vi "KH7008 Create Command String.vi"(8 "error in (no error)":errorcluster, 11 "Channel Params":T1={"Channel"=enum."Channel 2", "Gain"=enum."10x", "Bandwidth Filter"=enum."ON", "Shunt Resistor"=enum."50 Ohms", "Coupling"=enum."DC", "Input Config"=enum."Differential"}) -> (0 "error out":errorcluster, 3 "Command string":string)   [LabVIEW 2019, in "Inst.Krohn-Hite-7008.lvclass"]
uses:
  Inst.Krohn-Hite-7008.lvclass
  Typedefs/SetAll-Cluster.ctl
  Typedefs/Channel-Enum.ctl
  Typedefs/Gain-Enum.ctl
  Typedefs/Filter-Enum.ctl
  Typedefs/Shunt-Enum.ctl
  Typedefs/Coupling-Enum.ctl
  Typedefs/Input Configuration-Enum.ctl
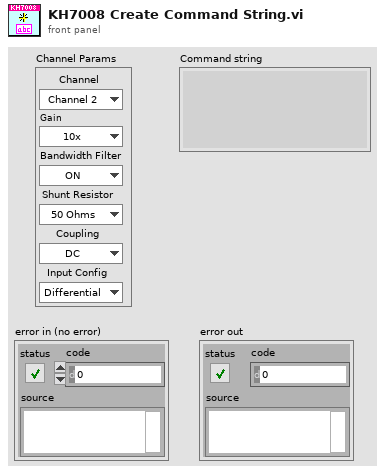
[diagram p1: front panel]
types:
  T1 = typedef "Inst.Krohn-Hite-7008.lvclass/SetAll-Cluster.ctl" = cluster{"Channel":T2, "Gain":T3, "Bandwidth Filter":T4, "Shunt Resistor":T5, "Coupling":T6, "Input Config":T7}
  T2 = typedef "Inst.Krohn-Hite-7008.lvclass/Channel-Enum.ctl" = enum16{"Channel 1", "Channel 2", "Channel 3", "Channel 4", "Channel 5", "Channel 6", "Channel 7", "Channel 8"}
  T3 = typedef "Inst.Krohn-Hite-7008.lvclass/Gain-Enum.ctl" = enum16{"1x", "10x", "100x", "1000x"}
  T4 = typedef "Inst.Krohn-Hite-7008.lvclass/Filter-Enum.ctl" = enum16{"OFF", "ON"}
  T5 = typedef "Inst.Krohn-Hite-7008.lvclass/Shunt-Enum.ctl" = enum16{"Open", "50 Ohms", "500 Ohms", "5k Ohms", "50k Ohms", "10M Ohm"}
  T6 = typedef "Inst.Krohn-Hite-7008.lvclass/Coupling-Enum.ctl" = enum16{"AC", "DC"}
  T7 = typedef "Inst.Krohn-Hite-7008.lvclass/Input Configuration-Enum.ctl" = enum16{"Ground", "SE+ (-gnd)", "SE- (+gnd)", "Differential"}
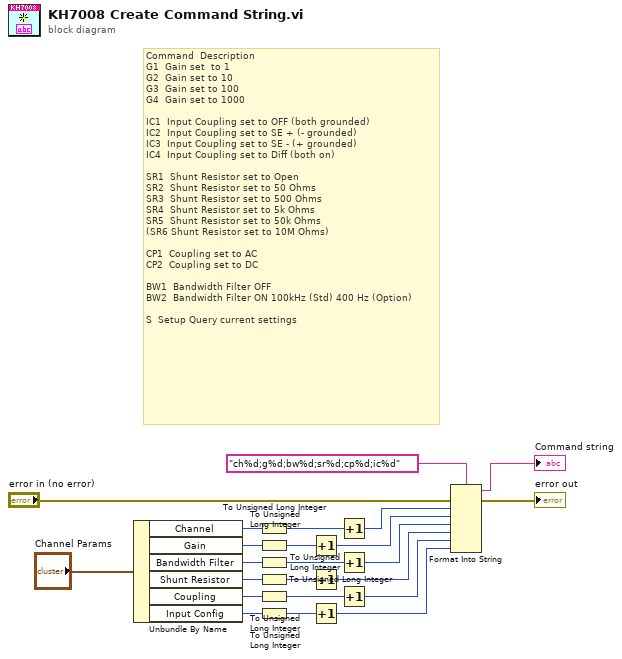
[diagram p0: block diagram]
diagram:
  # "Command  Description \nG1  Gain set  to 1 \nG2  Gain set to 10 \nG3  Gain set to 100 \nG4  Gain set to 1000 \n   \nIC1  Input Coupling set to OFF (both grounded) \nIC2  Input Coupling set to SE + (- grounded) \nIC3  Input Coupling set to SE - (+ grounded) \nIC4  Input Coupling set to Diff (both on) \n   \nSR1  Shunt Resistor set to Open \nSR2  Shunt Resistor set to 50 Ohms \nSR3  Shunt Resistor set to 500 Ohms \nSR4  Shunt Resistor set to 5k Ohms \nSR5  Shunt Resistor set to 50k Ohms \n(SR6 Shunt Resistor set to 10M Ohms)\n   \nCP1  Coupling set to AC \nCP2  Coupling set to DC \n   \nBW1  Bandwidth Filter OFF \nBW2  Bandwidth Filter ON 100kHz (Std) 400 Hz (Option)\n   \nS  Setup Query current settings"
  n1 = Unbundle By Name("Channel Params") -> ("Channel"=w6:T2, "Gain"=w5:T3, "Bandwidth Filter"=w4:T4, "Shunt Resistor"=w3:T5, "Coupling"=w2:T6, "Input Config"=w1:T7)
  n2 = To Unsigned Long Integer(number=w6) -> (unsigned 32bit integer=w15:u32)
  n3 = To Unsigned Long Integer(number=w5) -> (unsigned 32bit integer=w16:u32)
  n4 = To Unsigned Long Integer(number=w4) -> (unsigned 32bit integer=w17:u32)
  n5 = To Unsigned Long Integer(number=w3) -> (unsigned 32bit integer=w18:u32)
  n6 = To Unsigned Long Integer(number=w2) -> (unsigned 32bit integer=w19:u32)
  n7 = To Unsigned Long Integer(number=w1) -> (unsigned 32bit integer=w20:u32)
  n8 = Increment(x=w16) -> (x+1=w10:u32)
  n9 = Increment(x=w18) -> (x+1=w11:u32)
  n10 = Increment(x=w20) -> (x+1=w14:u32)
  n11 = Increment(x=w15) -> (x+1=w9:u32)
  n12 = Increment(x=w17) -> (x+1=w12:u32)
  n13 = Increment(x=w19) -> (x+1=w13:u32)
  n14 = Format Into String(format string="ch%d;g%d;bw%d;sr%d;cp%d;ic%d", error in="error in (no error)", w9, w10, w12, w11, w13, w14) -> (resulting string=→"Command string":string, error out=→"error out":errorcluster)  [unwired: 1 in]
